vi "PDE_Mtrx x Tridiag MtrxT.vi"(8 "X":dbl[][](array[numeric]), 9 "Super Diag":dbl[](array[numeric]), 10 "Diag":dbl[](array[numeric]), 11 "Sub Diag":dbl[](array[numeric])) -> (3 "X x MtrxT":dbl[][](array[numeric]))   [LabVIEW 2017, in "NI_PDE.lvlib"]
uses:
  <vilib>/gmath/NI_PDE.lvlib
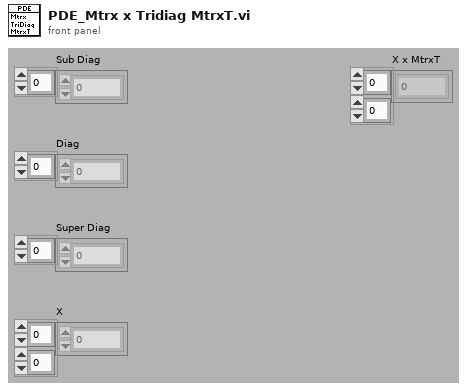
[diagram p1: front panel]
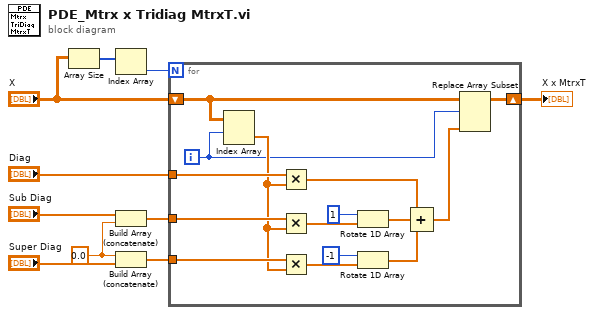
[diagram p0: block diagram]
diagram:
  w10 = 0.0
  n1 = Array Size(array="X") -> (size(s)=w5:i32[])
  n2 = Index Array(array=w5) -> (element=w3:i32)  [unwired: 1 in]
  n3 = Build Array (concatenate)("Sub Diag", w10) -> (w9:dbl[])
  n4 = Build Array (concatenate)(w10, "Super Diag") -> (w8:dbl[])
  n5 = for {
    N: w3 -> [_]
    tunnel: w9 -> [w25]
    tunnel: w8 -> [w24]
    tunnel: "Diag" -> [w23]
    shift-right: [w13] -> w6
    shift-left: "X" -> [w14]
    i -> [w11]
    n6 = Index Array(array=w14, index (row)=w11) -> (element=w15:dbl[])  [unwired: 1 in]
    n7 = Multiply(x=w23, y=w15) -> (x*y=w22:dbl[])
    n8 = Multiply(x=w25, y=w15) -> (x*y=w21:dbl[])
    n9 = Multiply(x=w24, y=w15) -> (x*y=w17:dbl[])
    n10 = Rotate 1D Array(1:w21, 2:1 ("n")) -> (0:w20:dbl[])
    n11 = Rotate 1D Array(1:w17, 2:-1 ("n")) -> (0:w16:dbl[])
    n12 = Compound Arithmetic op=ADD(w22, w20, w16) -> (w12:dbl[])
    n13 = Replace Array Subset(array=w14, new element=w12, index (row)=w11) -> (w13:dbl[][])  [unwired: 1 in]
  }
  "X x MtrxT" <- w6
